vi "fit_fix height and width.vi"() -> ()   [LabVIEW 2016] (continued)
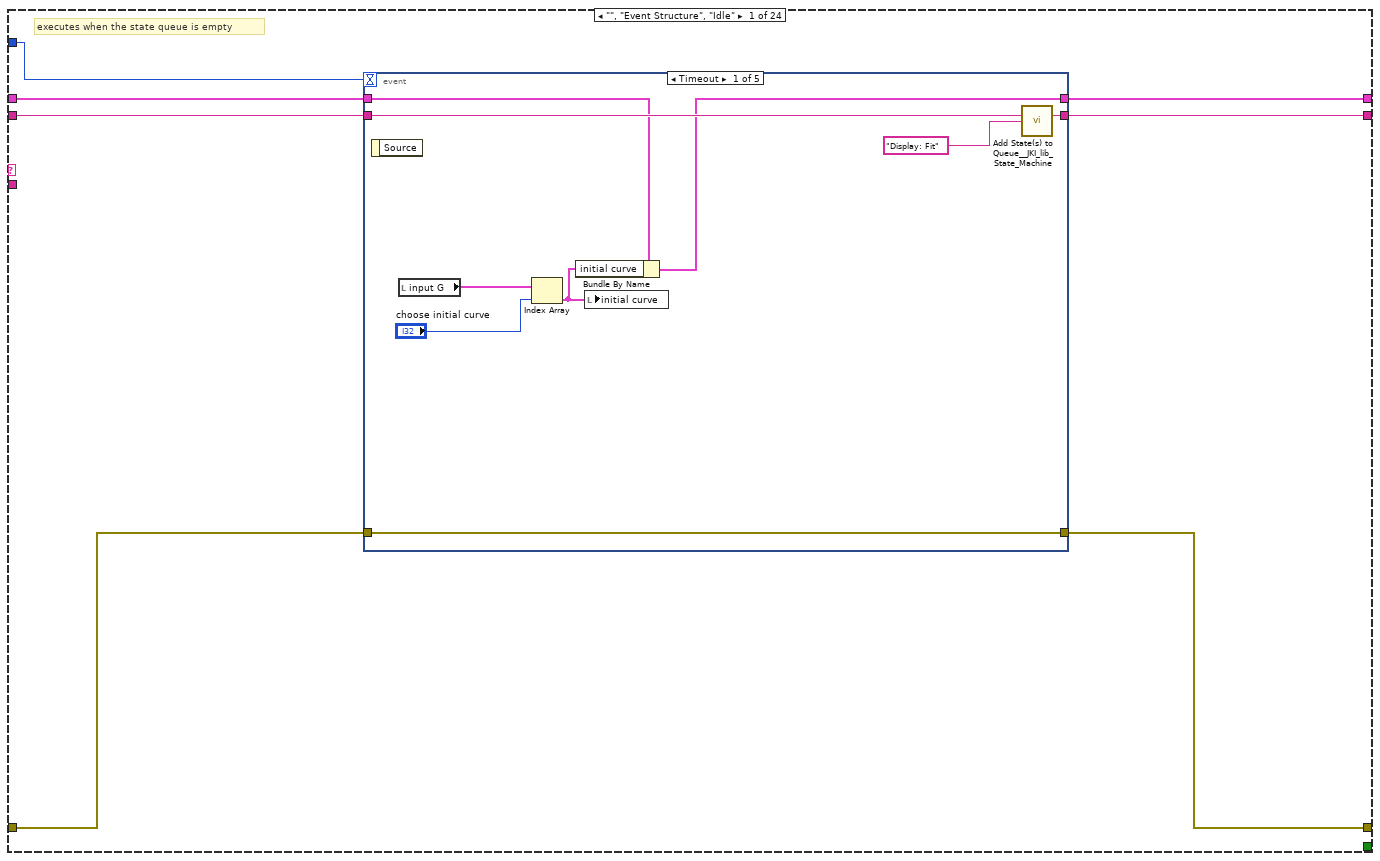
[diagram p3: hidden frame]
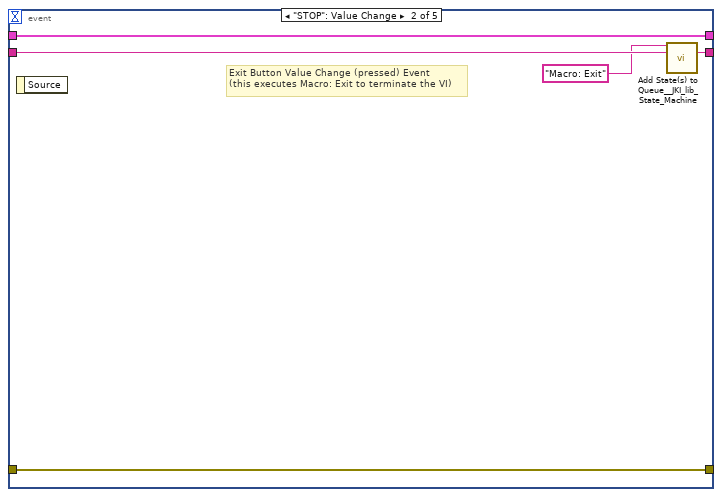
[diagram p4: hidden frame]
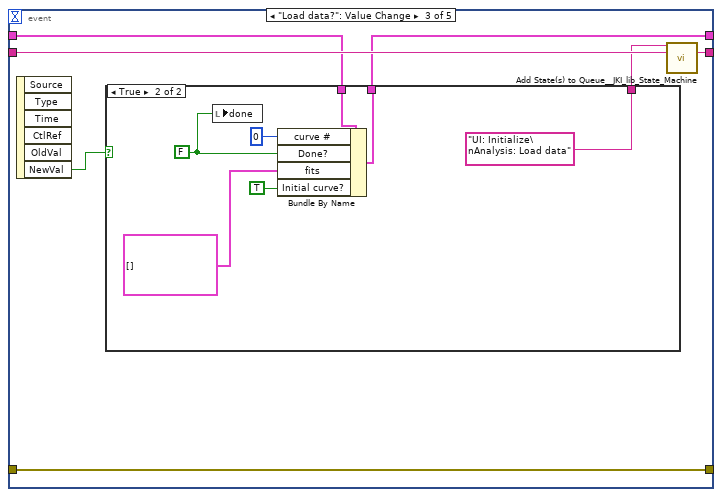
[diagram p5: hidden frame]
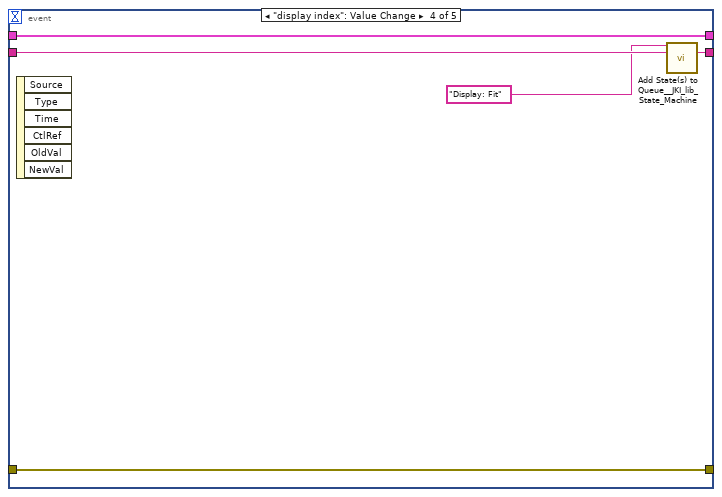
[diagram p7: hidden frame]
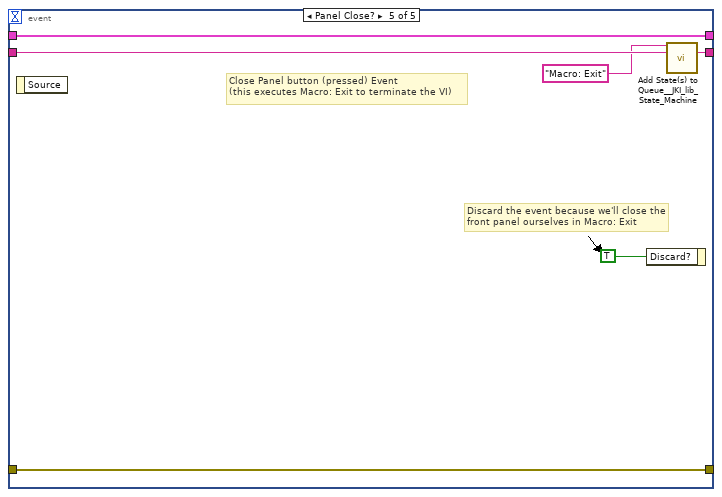
[diagram p8: hidden frame]
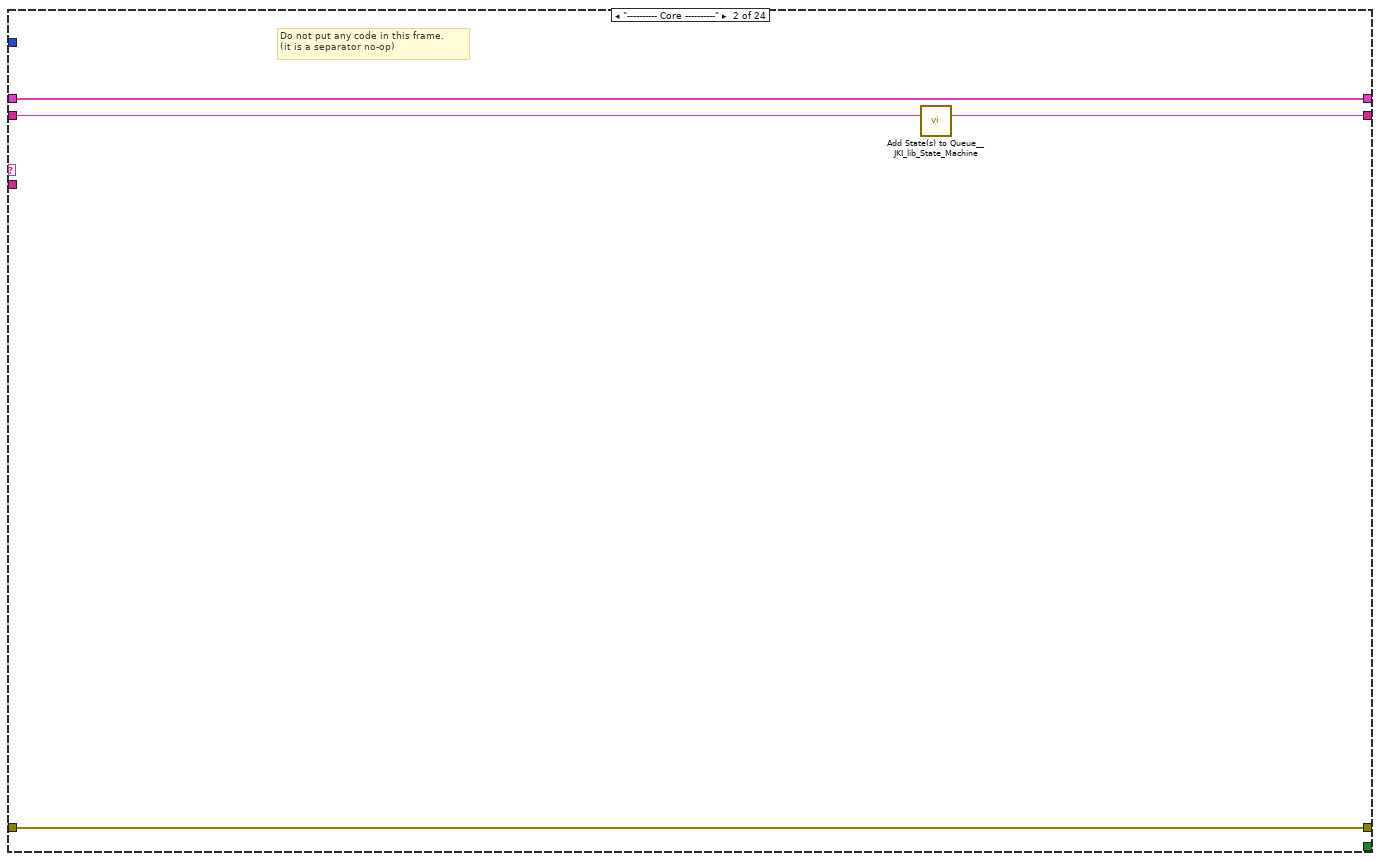
[diagram p9: hidden frame]
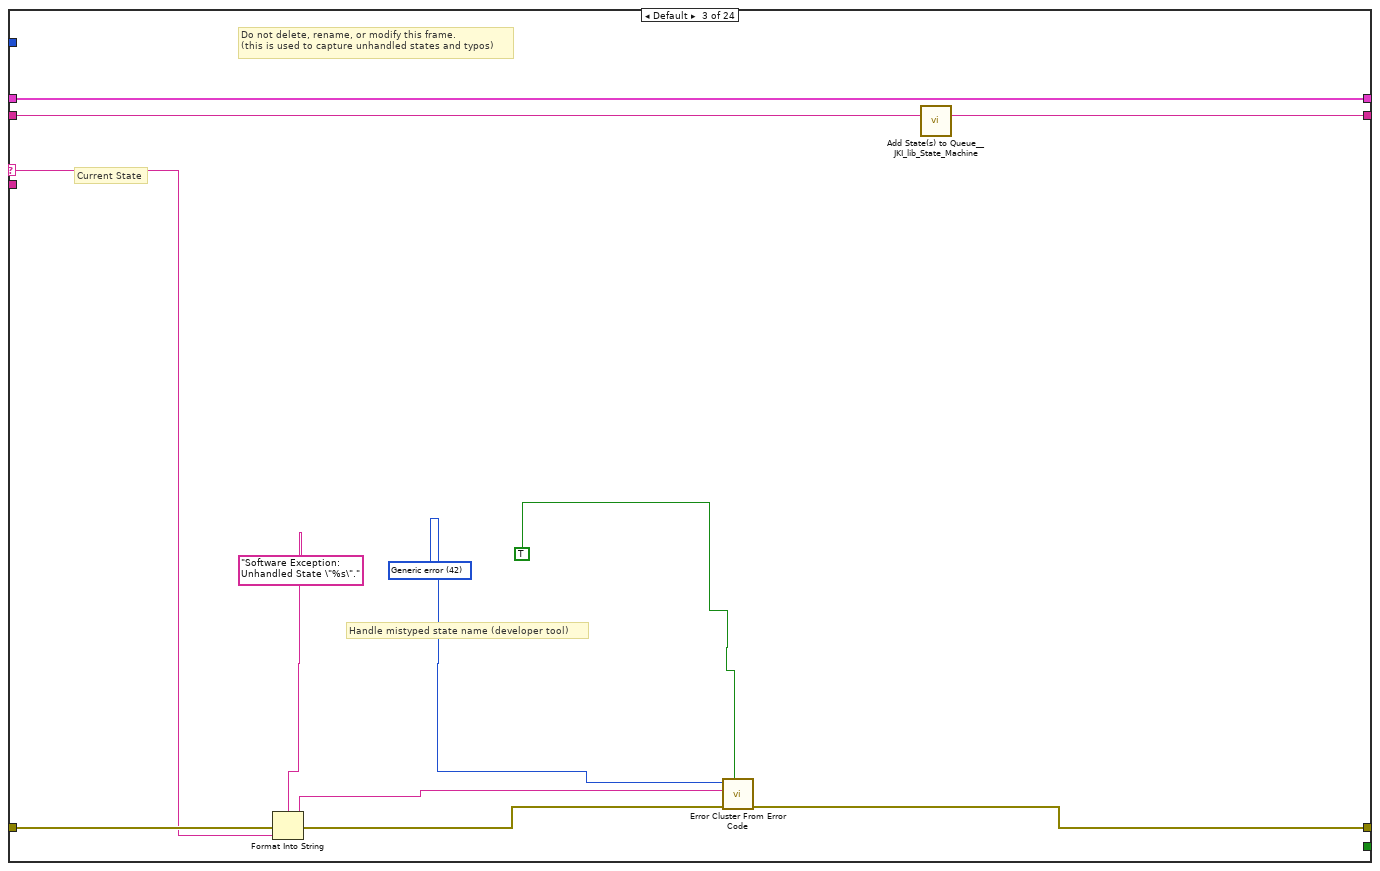
[diagram p10: hidden frame]
        n68 = call <vilib>:"Add State(s) to Queue__JKI_lib_State_Machine.vi"("State(s) in Front (\"\")"=w206, "State(s) in (\"\")"=w215) -> ("States Out"=w214:string)  [unwired: 13 in]
      }
      frame "---------- Analysis ----------" {
        # "Template Separator\n(You can make a copy of, or modify, this frame)"
        n69 = call <vilib>:"Add State(s) to Queue__JKI_lib_State_Machine.vi"("State(s) in (\"\")"=w219) -> ("States Out"=w218:string)  [unwired: 14 in]
      }
      frame "Analysis: Load data" {
        # "Load data and step through curves for fitting"
        n70 = local read "input G"() -> (w230:cluster{dbl[], dbl[]}[])
        n71 = Unbundle By Name(w243) -> ("curve #"=w229:i32, "fit iteration"=w225:i32, "Initial curve?"=w233:bool)
        "curve #" <- w229
        n72 = Array Size(array=w230) -> (size(s)=w228:i32)
        n73 = Decrement(x=w228) -> (x-1=w227:i32)
        n74 = case shown="True" "Restrict G?" {
          tunnel: w230 -> [w249 w251]
          tunnel: [w249 w250] -> w242
          frame False {
          }
          frame True {
            n75 = for {
              tunnel: w251 -> [w259] mode=indexing
              tunnel: [w252] -> w250 mode=indexing
              n76 = Unbundle(w259) -> (w257:dbl[], w256:dbl[])
              n77 = Threshold 1D Array(2:"Max G", 3:w256) -> (0:w255:dbl)  [unwired: 1 in]
              n78 = Array Subset(array=w256, length=w255) -> (w253:dbl[])  [unwired: 1 in]
              n79 = Array Subset(array=w257, length=w255) -> (w254:dbl[])  [unwired: 1 in]
              n80 = Bundle(w254, w253) -> (w252:cluster{dbl[], dbl[]})  [unwired: 1 in]
            }
          }
        }
        n81 = Equal?(x=w229, y=w227) -> (x = y?=w226:bool)
        n82 = Equal?(x=w225, y=0) -> (x = y?=w223:bool)
        n83 = And(x=w226, y=w223) -> (x .and. y?=w222:bool)
        n84 = local read "choose initial curve"() -> (w232:i32)
        n85 = case shown="True" w222 {
          frame False {
          }
          frame True {
            n86 = call <vilib>:"Beep.vi"() -> ()  [unwired: 12 in]
          }
        }
        n87 = Select(t=w232, s=w233, f=w229) -> (s? t:f=w231:i32)
        n88 = Index Array(array=w242, index=w231) -> (element=w234:cluster{dbl[], dbl[]})
        n89 = local write "Single G"(w234) -> ()
        n90 = local write "Restricted G"(w242) -> ()
        n91 = Unbundle(w234) -> (w240:dbl[])  [unwired: 1 out]
        n92 = Array Max & Min(array=w240) -> (max value=w241:dbl)  [unwired: 3 out]
        n93 = Round Toward -Infinity(1:w241) -> (0:w221:dbl)
        n94 = Add(x=w221, y=w225) -> (x+y=w239:dbl)
        n95 = Bundle By Name(cluster=w243, "All G"=w242, "Single G curve"=w234, "model step #"=w239) -> (w245:T5)
        n96 = Equal?(x=0, y=w225) -> (x = y?=w237:bool)
        n97 = Select(t="Analysis: find peaks" ("State(s) at Back (\"\")"), s=w237, f="Analysis: Initial Parameters" ("State(s) at Back (\"\")")) -> (s? t:f=w220:string)
        n98 = call <vilib>:"Add State(s) to Queue__JKI_lib_State_Machine.vi"("State(s) in Front (\"\")"=w220, "State(s) in (\"\")"=w248) -> ("States Out"=w247:string)  [unwired: 13 in]
      }
      frame "Analysis: find peaks" {
        # "Fid peak locations to help constrain step position inital parameters"
        n99 = Unbundle By Name(w271) -> ("Single G curve"=w272:cluster{"Single G curve":dbl[], dbl[]})
        n100 = call <userlib>:"differential.vi"("Numeric"="derivative \nfor peak initial conditions", "dy/dx vs x"=TRUE, "A vs B 2"=w272) -> ("A vs B 3"=w267:T8)  [unwired: 1 in]
        n101 = Unbundle(w267) -> ("Decimated Array"=w263:dbl[], "Decimated Array"=w266:dbl[])
        n102 = call <vilib>:"Peak Detector.vi"("width"="derivative peak width", "threshold"="derivative peak threshold", "X"=w266) -> ("Locations"=w262:dbl[])  [unwired: 4 in, 4 out]
        "Locations index" <- w262
        n103 = for {
          N -> [w276]
          tunnel: w263 -> [w279]
          tunnel: w262 -> [w278] mode=indexing
          tunnel: [w277] -> w261 mode=indexing
          tunnel: [w276] -> _ mode=indexing
          n104 = Interpolate 1D Array(1:w278, 2:w279) -> (0:w277:dbl)
        }
        "Locations" <- w261
        n105 = call <vilib>:"Add State(s) to Queue__JKI_lib_State_Machine.vi"("State(s) in Front (\"\")"="Analysis: Initial Parameters" ("State(s) at Back (\"\")"), "State(s) in (\"\")"=w275) -> ("States Out"=w274:string)  [unwired: 13 in]
        n106 = Bundle By Name(cluster=w271, "Locations index"=w262, "Locations"=w261) -> (w270:T5)
      }
      frame "Analysis: Initial Parameters" {
        # "Create initial parameter and parameter bound arrays"
        n107 = Unbundle By Name(w306) -> ("Initial Best Fit"=w297:dbl[], "Initial curve?"=w288:bool, "model step #"=w301:i32, "Single G curve"=w309:cluster{"Single G curve":dbl[], dbl[]}, "Locations index"=w308:dbl[], "Locations"=w307:dbl[], "Best Fit Parameters"=w292:dbl[][], "residues"=w291:dbl[], "curve #"=w281:i32)
        n108 = case shown="True" "fix step width?" {
          tunnel: [w315 w316] -> w296
          tunnel: [w314 w316] -> w295
          tunnel: ["step width?" w316] -> w284
          tunnel: w281 -> [_ w324]
          frame False {
            n109 = local read "step width max"() -> (w315:dbl)
            n110 = local read "step width min"() -> (w314:dbl)
          }
          frame True {
            n111 = local read "B multiplier"() -> (w323:dbl)
            n112 = local read "B offset"() -> (w321:dbl)
            n113 = Multiply(x=w324, y=w323) -> (x*y=w322:dbl)
            n114 = Add(x=w322, y=w321) -> (x+y=w319:dbl)
            n115 = Multiply(x=w319, y="fix width slope") -> (x*y=w317:dbl)
            n116 = Add(x=w317, y="fix width intercept") -> (x+y=w316:dbl)
          }
        }
        n117 = Array Size(array=w291) -> (size(s)=w290:i32)
        n118 = Unbundle(w309) -> ("Single G curve"=w302:dbl[], w303:dbl[])
        n119 = Select(t=w288, s="fit inital parameters?", f=TRUE) -> (s? t:f=w287:bool)
        n120 = Decrement(x=w290) -> (x-1=w289:i32)
        n121 = case shown="True" w287 {
          tunnel: w308 -> [w339 w400]
          tunnel: w307 -> [w338 w399]
          tunnel: [w347 w398] -> w305
          tunnel: w303 -> [w341 w397]
          tunnel: w302 -> [w344 w396]
          tunnel: w301 -> [w351 w395]
          tunnel: [w337 w394] -> w300
          tunnel: [w345 w393] -> w299
          tunnel: w297 -> [w348 _]
          tunnel: w296 -> [w336 w392]
          tunnel: w295 -> [w335 w391]
          tunnel: "step height max" -> [w334 w390]
          tunnel: "step height min" -> [w333 w389]
          tunnel: w292 -> [w332 _]
          tunnel: w289 -> [w331 _]
          tunnel: "one width?" -> [_ w388]
          tunnel: w284 -> [_ w387]
          frame False {
            w346 = dbl[] []
            n122 = Index Array(array=w332, index (row)=w331) -> (element=w330:dbl[])  [unwired: 1 in]
            n123 = Array Max & Min(array=w344) -> (max value=w343:dbl, min value=w342:dbl)  [unwired: 2 out]
            n124 = call-poly <userlib>:"Filter 1D Array__ogtk.vi"("items to filter"=0.0, "array"=w348) -> ("filtered array"=w352:dbl[])  [unwired: 4 in, 1 out]
            n125 = Decimate 1D Array(w330) -> (w328:dbl[])  [unwired: 2 out]
            n126 = Multiply(x=w328, y="Max position %") -> (x*y=w326:dbl[])
            n127 = Multiply(x=w328, y="Min position %") -> (x*y=w325:dbl[])
            n128 = Decimate 1D Array(w352) -> (w350:dbl[], w349:dbl[])  [unwired: 1 out]
            n129 = for {
              N: w351 -> [_]
              tunnel: w350 -> [w386]
              tunnel: w349 -> [w385]
              shift-right: [w383] -> w347
              shift-left: dbl[] [] -> [w384]
              shift-right: [w381] -> w345
              shift-left: w346 -> [w382]
              shift-right: [w379] -> w337
              shift-left: w346 -> [w380]
              tunnel: w343 -> [w371]
              tunnel: w342 -> [w368]
              tunnel: w341 -> [w378]
              tunnel: w339 -> [w377]
              tunnel: w338 -> [w375]
              tunnel: w336 -> [w360]
              tunnel: w335 -> [w359]
              tunnel: w334 -> [w362]
              tunnel: w333 -> [w361]
              tunnel: w326 -> [w367]
              tunnel: w325 -> [w365]
              i -> [w364]
              n130 = Index Array(array=w367, index=w364) -> (element=w366:dbl)
              n131 = Index Array(array=w365, index=w364) -> (element=w363:dbl)
              n132 = Index Array(array=w386, index=w364) -> (element=w356:dbl)
              n133 = Index Array(array=w385, index=w364) -> (element=w372:dbl)
              n134 = Threshold 1D Array(2:w364, 3:w378) -> (0:w376:dbl)  [unwired: 1 in]
              n135 = call "compare if zero.vi"("if zero out"=w368, "Numeric"=w363) -> ("out"=w369:dbl)  [unwired: 5 in]
              n136 = call "compare if zero.vi"("if zero out"=w362, "Numeric"=w356) -> ("out"=w358:dbl)  [unwired: 5 in]
              n137 = call "compare if zero.vi"("if zero out"=w371, "Numeric"=w366) -> ("out"=w370:dbl)  [unwired: 5 in]
              n138 = call "Search 1D Array for Nearest LV2012 NIVerified.vi"("desired element"=w376, "1D Array"=w377) -> ("closest index"=w374:i32)  [unwired: 8 in, 1 out]
              n139 = call "compare if zero.vi"("if zero out"=w360, "Numeric"=w372) -> ("out"=w355:dbl)  [unwired: 5 in]
              n140 = call "compare if zero.vi"("if zero out"=w361, "Numeric"=w356) -> ("out"=w357:dbl)  [unwired: 5 in]
              n141 = call "compare if zero.vi"("if zero out"=w359, "Numeric"=w372) -> ("out"=w354:dbl)  [unwired: 5 in]
              n142 = Index Array(array=w375, index=w374) -> (element=w373:dbl)
              n143 = Build Array (concatenate)(w382, w358, w370, w355) -> (w381:dbl[])
              n144 = Build Array (concatenate)(w380, w357, w369, w354) -> (w379:dbl[])
              n145 = Build Array (concatenate)(w384, w356, w373, w372) -> (w383:dbl[])
            }
          }
          frame True {
            n146 = case shown="True" w388 {
              tunnel: w400 -> [w418 w453]
              tunnel: w399 -> [w417 w452]
              tunnel: [w416 w451] -> w398
              tunnel: w397 -> [w415 w450]
              tunnel: w396 -> [w414 w448]
              tunnel: w395 -> [w411 w445]
              tunnel: [w410 w444] -> w394
              tunnel: [w409 w443] -> w393
              tunnel: w392 -> [w404 w441]
              tunnel: w391 -> [w402 w440]
              tunnel: w390 -> [w408 w439]
              tunnel: w389 -> [w407 w438]
              tunnel: w387 -> [w406 w437]
              frame True {
                n147 = Array Max & Min(array=w414) -> (max value=w413:dbl, min value=w412:dbl)  [unwired: 2 out]
                n148 = Build Array(w406) -> (w405:dbl[])
                n149 = Build Array(w404) -> (w403:dbl[])
                n150 = Build Array(w402) -> (w401:dbl[])
                n151 = for {
                  N: w411 -> [_]
                  tunnel: w415 -> [w436]
                  shift-right: [w428] -> w416
                  shift-left: w405 -> [w429]
                  tunnel: w418 -> [w434]
                  tunnel: w417 -> [w432]
                  shift-right: [w426] -> w409
                  shift-left: w403 -> [w427]
                  shift-right: [w425] -> w410
                  shift-left: w401 -> [w424]
                  tunnel: w413 -> [w423]
                  tunnel: w412 -> [w421]
                  tunnel: w404 -> [_]
                  tunnel: w402 -> [_]
                  tunnel: w408 -> [w420]
                  tunnel: w407 -> [w419]
                  i -> [w435]
                  n152 = Threshold 1D Array(2:w435, 3:w436) -> (0:w433:dbl)  [unwired: 1 in]
                  n153 = call "Search 1D Array for Nearest LV2012 NIVerified.vi"("desired element"=w433, "1D Array"=w434) -> ("closest index"=w422:i32)  [unwired: 8 in, 1 out]
                  n154 = Index Array(array=w432, index=w422) -> (element=w430:dbl)
                  n155 = Build Array (concatenate)(w429, 1.0 ("element"), w430) -> (w428:dbl[])
                  n156 = Build Array (concatenate)(w427, w420, w423) -> (w426:dbl[])
                  n157 = Build Array (concatenate)(w424, w419, w421) -> (w425:dbl[])
                }
              }
              frame False {
                w442 = dbl[] []
                n158 = Array Max & Min(array=w448) -> (max value=w447:dbl, min value=w446:dbl)  [unwired: 2 out]
                n159 = for {
                  N: w445 -> [_]
                  tunnel: w450 -> [w474]
                  shift-right: [w466] -> w451
                  shift-left: dbl[] [] -> [w467]
                  tunnel: w453 -> [w472]
                  tunnel: w452 -> [w470]
                  shift-right: [w464] -> w443
                  shift-left: w442 -> [w465]
                  shift-right: [w463] -> w444
                  shift-left: w442 -> [w462]
                  tunnel: w447 -> [w461]
                  tunnel: w446 -> [w459]
                  tunnel: w441 -> [w458]
                  tunnel: w440 -> [w457]
                  tunnel: w439 -> [w456]
                  tunnel: w438 -> [w455]
                  tunnel: w437 -> [w454]
                  i -> [w473]
                  n160 = Threshold 1D Array(2:w473, 3:w474) -> (0:w471:dbl)  [unwired: 1 in]
                  n161 = call "Search 1D Array for Nearest LV2012 NIVerified.vi"("desired element"=w471, "1D Array"=w472) -> ("closest index"=w460:i32)  [unwired: 8 in, 1 out]
                  n162 = Index Array(array=w470, index=w460) -> (element=w468:dbl)
                  n163 = Build Array (concatenate)(w467, 1.0 ("element"), w468, w454) -> (w466:dbl[])
                  n164 = Build Array (concatenate)(w465, w456, w461, w458) -> (w464:dbl[])
                  n165 = Build Array (concatenate)(w462, w455, w459, w457) -> (w463:dbl[])
                }
              }
            }
          }
        }
        "Initial Parameters" <- w305
        n166 = Bundle(w300, w299) -> (w298:cluster{dbl[], dbl[]})  [unwired: 1 in]
        n167 = call <vilib>:"Add State(s) to Queue__JKI_lib_State_Machine.vi"("State(s) in Front (\"\")"="Analysis: Fit" ("State(s) at Back (\"\")"), "State(s) in (\"\")"=w312) -> ("States Out"=w311:string)  [unwired: 13 in]
        n168 = Bundle By Name(cluster=w306, "Initial Parameters"=w305, "parameter bounds"=w298, "one width?"="one width?") -> (w304:T5)
      }
      frame "Analysis: Fit" {
        (unwired) errorcluster {"status"=FALSE, "code"=0, "source"=""} ("error out")
        # "increase termination conditions \nif there is a max iteration error"
        # "Fit data"
        n169 = Unbundle By Name(w511) -> ("termination"=w498:cluster{"max iteration":i32, "tolerance":dbl}, "intermediate fits"=w501:cluster{dbl[], dbl[]}[], "Single G curve"=w508:cluster{"Single G curve":dbl[], dbl[]}, "Initial Parameters"=w515:dbl[], "Intermediate Best Fit"=w509:dbl[][], "intermediate residues"=w504:dbl[], "termination"=w506:cluster{"max iteration":i32, "tolerance":dbl}, "parameter bounds"=w507:T6, "Intermediate delta"=w484:dbl[][])
        "termination" <- w506
        n170 = case shown="\"normal tanh\", Default" "fit vi path" {
          tunnel: [path "C:/user/megan/hg/levylab_user_megan/data analysis/pascal fitting/subVI/LM model function and gradient_step.vi" ("vi path") path "C:/user/megan/hg/levylab_user_megan/data analysis/pascal fitting/subVI/LM model function_1 width.vi" ("vi path")] -> w485
          frame "normal tanh", Default {
          }
          frame "tanh w/ 1 width" {
          }
        }
        n171 = Unbundle(w508) -> ("Single G curve"=w481:dbl[], w482:dbl[])
        n172 = Open VI Reference(type specifier VI Refnum (for type only)=refnum<vi> refnum, vi path=w485) -> (vi reference=w512:refnum<vi>)  [unwired: 4 in, 1 out]
        n173 = call-by-ref "?"(reference=w512, "X"=w481, "a"=w515) -> (reference out=w479:refnum<vi>)  [unwired: 3 in, 4 out]
        n174 = Unbundle(w498) -> ("max iteration"=w497:i32, "tolerance"=w496:dbl)
        n175 = call-poly <vilib>:"Constrained Nonlinear Curve Fit.vi"("Y"=w482, "f(x,a)"=w479, "X"=w481, "initial parameters"=w515, "error in (no error)"=w510, "termination"=w506, "parameter bounds"=w507, "method"="method") -> ("best nonlinear fit"=w491:dbl[], "best fit parameters"=w480:dbl[], "residue"=w487:dbl, "error out"=w477:errorcluster)  [unwired: 2 in, 2 out]
        n176 = call <vilib>:"Goodness of Fit.vi"("Best Fit"=w491, "Y"=w482) -> ("RMSE"=→"RMSE":dbl, "R-square"=→"R-square":dbl, "SSE"=→"SSE":dbl)  [unwired: 6 in, 1 out]
        n177 = disable-structure shown="Disabled" {
          disable-tunnel: w482 -> [w523 _]
          disable-tunnel: w481 -> [w522 _]
          disable-tunnel: w480 -> [w521 _]
          disable-tunnel: w479 -> [w520 _]
          disable-tunnel: [w519 _] -> w478
          disable-tunnel: w477 -> [w518 _]
          frame Disabled {
            n178 = call <vilib>:"Nonlinear Curve Fit Intervals.vi"("Y"=w523, "f(x,a)"=w520, "X"=w522, "best fit parameters"=w521, "error in (no error)"=w518) -> ("delta best fit parameters"=w519:dbl[])  [unwired: 7 in, 3 out]
          }
          frame Enabled {
          }
        }
        n179 = Bundle("Single G curve"=w481, "best nonlinear fit"=w491) -> (w502:T9)  [unwired: 1 in]
        n180 = Equal?(x=errorcluster {"status"=TRUE, "code"=-23026, "source"="maximum iterations exceeded"} ("error out"), y=w477) -> (x = y?=w499:bool)
        n181 = case shown="True" w499 {
          tunnel: w509 -> [w541 w553]
          tunnel: w480 -> [w540 _]
          tunnel: [w539 w553] -> w505
          tunnel: w504 -> [w538 w552]
          tunnel: w487 -> [w537 _]
          tunnel: [w536 w552] -> w503
          tunnel: w502 -> [w535 _]
          tunnel: [w534 w551] -> w500
          tunnel: w501 -> [w533 w551]
          tunnel: w497 -> [w532 w547]
          tunnel: w496 -> [w531 w548]
          tunnel: [w531 w546] -> w494
          tunnel: [w532 w545] -> w495
          tunnel: ["Analysis: Iterate" "Analysis: Fit"] -> w475
          tunnel: w477 -> [w527 _]
          tunnel: [w527 errorcluster {"status"=FALSE, "code"=0, "source"=""} ("error out")] -> w493
          tunnel: w484 -> [w529 w542]
          tunnel: [w528 w542] -> w483
          tunnel: w480 -> [_ _]
          tunnel: w481 -> [_ _]
          tunnel: w482 -> [_ _]
          tunnel: w479 -> [_ _]
          tunnel: w478 -> [w526 _]
          frame False {
            n182 = Build Array (concatenate)(w541, w540) -> (w539:dbl[][])
            n183 = Build Array (concatenate)(w538, w537) -> (w536:dbl[])
            n184 = Build Array (concatenate)(w529, w526) -> (w528:dbl[][])
            n185 = Insert Into Array(array=w533, new element=w535) -> (w534:cluster{dbl[], dbl[]}[])  [unwired: 1 in]
          }
          frame True {
            n186 = Multiply(x=w548, y=2.0) -> (x*y=w546:dbl)
            n187 = Add(x=w547, y=200) -> (x+y=w545:i32)
          }
        }
        "intermediate residues" <- w503
        "Intermediate Best Fit" <- w505
        n188 = Bundle By Name(cluster=w511, "termination.max iteration"=w495, "termination.tolerance"=w494, "intermediate fits"=w500, "Intermediate Best Fit"=w505, "intermediate residues"=w503, "Intermediate delta"=w483) -> (w514:T5)
        n189 = call <vilib>:"Add State(s) to Queue__JKI_lib_State_Machine.vi"("State(s) in Front (\"\")"=w475, "State(s) in (\"\")"=w517) -> ("States Out"=w516:string)  [unwired: 13 in]
      }
      frame "Analysis: Iterate" {
        # "Iterate curve # and fit iteration #\nincrement fit iteration\nif fit iteration = 3, set to 0 and increment curve #\nif curve # is greater than the total # of curves end fitting"
        n190 = Unbundle By Name(w590) -> ("curve #"=w585:i32, "All G"=w584:cluster{dbl[], dbl[]}[], "fit iteration"=w588:i32, "Best Fit Parameters"=w579:dbl[][], "Intermediate Best Fit"=w581:dbl[][], "intermediate residues"=w580:dbl[], "residues"=w573:dbl[], "Intermediate delta"=w559:dbl[][], "delta best fit"=w556:dbl[][], "fits"=w560:cluster{dbl[], dbl[]}[], "intermediate fits"=w575:cluster{dbl[], dbl[]}[], "Initial curve?"=w571:bool, "Initial Best Fit"=w569:dbl[], "All locations"=w567:dbl[][], "Locations"=w568:dbl[], "Fit steps"=w564:i32[], "model step #"=w563:i32)
        n191 = Increment(x=w588) -> (x+1=w587:i32)
        n192 = case shown="4" w587 {
          selector: w587 -> [w608 _]
          tunnel: [w608 0] -> w586
          tunnel: w585 -> [w607 w624]
          tunnel: w584 -> [_ w651]
          tunnel: [w607 w647] -> w583
          tunnel: ["Analysis: Load data" w646] -> w554
          tunnel: w581 -> [w603 w622]
          tunnel: w580 -> [w605 w645]
          tunnel: w579 -> [w604 w644]
          tunnel: [w604 w643] -> w576
          tunnel: [w603 w612] -> w578
          tunnel: [w605 dbl[] [] ("residues")] -> w577
          tunnel: w560 -> [w602 w640]
          tunnel: w575 -> [w601 w641]
          tunnel: [w602 w638] -> w574
          tunnel: [w601 cluster{dbl[], dbl[]}[] [] ("intermediate fits")] -> w558
          tunnel: w573 -> [w600 w636]
          tunnel: [w600 w634] -> w572
          tunnel: w571 -> [w599 w632]
          tunnel: [w599 FALSE] -> w570
          tunnel: [w598 w631] -> w562
          tunnel: w569 -> [w598 w630]
          tunnel: w568 -> [_ w627]
          tunnel: w567 -> [w597 w628]
          tunnel: [w597 w626] -> w566
          tunnel: w564 -> [w596 w625]
          tunnel: [w596 w623] -> w565
          tunnel: w563 -> [_ _]
          tunnel: w559 -> [w595 w615]
          tunnel: [w595 w612] -> w557
          tunnel: w556 -> [w594 w613]
          tunnel: [w594 w611] -> w555
          frame 0, Default {
          }
          frame 4 {
            w612 = dbl[][] [] ("Intermediate Best Fit")
            n193 = Increment(x=w624) -> (x+1=w648:i32)
            n194 = Array Size(array=w651) -> (size(s)=w649:i32)
            n195 = Array Max & Min(array=w645) -> (min value=w635:dbl, min index (indices)=w614:i32)  [unwired: 2 out]
            n196 = Less?(x=w648, y=w649) -> (x < y?=w650:bool)
            n197 = Index Array(array=w641, index=w614) -> (element=w639:cluster{dbl[], dbl[]})
            n198 = Index Array(array=w622, index (row)=w614) -> (element=w618:dbl[])  [unwired: 1 in]
            n199 = Index Array(array=w615, index (row)=w614) -> (element=w610:dbl[])  [unwired: 1 in]
            n200 = case shown="True" w632 {
              tunnel: w618 -> [w654 w657]
              tunnel: [w655 w657] -> w631
              tunnel: w630 -> [w655 _]
              tunnel: [w654 w656] -> w629
              tunnel: w610 -> [w653 _]
              tunnel: [w653 w656] -> w609
              frame False {
              }
              frame True {
                w656 = dbl[] [] ("residues")
              }
            }
            n201 = case shown="True" w650 {
              tunnel: w648 -> [_ w660]
              tunnel: [0 w660] -> w647
              tunnel: ["Display: Fit" "Analysis: Load data"] -> w646
              frame False {
              }
              frame True {
              }
            }
            n202 = call-poly <userlib>:"Filter 1D Array__ogtk.vi"("items to filter"=0, "array"=w618) -> ("filtered array"=w617:dbl[])  [unwired: 4 in, 1 out]
            n203 = Build Array (concatenate)(w628, w627) -> (w626:dbl[][])
            n204 = Build Array (concatenate)(w636, w635) -> (w634:dbl[])
            n205 = Array Size(array=w617) -> (size(s)=w621:i32)
            n206 = Build Array (concatenate)(w640, w639) -> (w638:cluster{dbl[], dbl[]}[])
            n207 = Build Array (concatenate)(w613, w609) -> (w611:dbl[][])
            n208 = Divide(x=w621, y=3) -> (x/y=w619:dbl)
            n209 = Build Array (concatenate)(w644, w629) -> (w643:dbl[][])
            n210 = Build Array (concatenate)(w625, w619) -> (w623:dbl[])
          }
        }
        "Best Fit Parameters" <- w576
        "residues" <- w572
        "Initial Best Fit" <- w562
        "Fit steps" <- w565
        "delta best fit" <- w555
        n211 = call <vilib>:"Add State(s) to Queue__JKI_lib_State_Machine.vi"("State(s) in Front (\"\")"=w554, "State(s) in (\"\")"=w593) -> ("States Out"=w592:string)  [unwired: 13 in]
        n212 = local write "fits"(w574) -> ()
        n213 = call "parse best fit into string array.vi"("Initial Best Fit"=w562) -> ("concatenated string"=→"initial best fit":string)  [unwired: 10 in]
        n214 = Bundle By Name(cluster=w590, "curve #"=w583, "fit iteration"=w586, "termination"=cluster{"max iteration":i32, "tolerance":dbl} {"max iteration"=200, "tolerance"=1e-08}, "Best Fit Parameters"=w576, "Intermediate Best Fit"=w578, "intermediate residues"=w577, "residues"=w572, "Intermediate delta"=w557, "delta best fit"=w555, "intermediate fits"=w558, "fits"=w574, "Initial curve?"=w570, "Initial Best Fit"=w562, "All locations"=w566, "Fit steps"=w565) -> (w591:T5)
      }
      frame "----------Display-------------" {
        # "Your code here.\n(You can make a copy of, or modify, this frame)"
        n215 = call <vilib>:"Add State(s) to Queue__JKI_lib_State_Machine.vi"("State(s) in (\"\")"=w665) -> ("States Out"=w664:string)  [unwired: 14 in]
      }
      frame "Display: Fit" {
        # "place holder for B field values"
        # "extract and sort Vsg peak values"
        n216 = Unbundle By Name(w723) -> ("All G"=w721:cluster{dbl[], dbl[]}[], "fits"=w716:cluster{dbl[], dbl[]}[], "Best Fit Parameters"=w714:dbl[][], "residues"=w713:dbl[], "one width?"=w670:bool, "delta best fit"=w669:dbl[][])  [unwired: 1 out]
        n217 = Index Array(array=w713, index="display index") -> (element=→"Display residue":dbl)
        n218 = Array Size(array=w713) -> (size(s)=w712:i32)
        n219 = for {
          N: w712 -> [_]
          tunnel: [w804] -> w667 mode=indexing
          i -> [w806]
          n220 = local read "B multiplier"() -> (w802:dbl)
          n221 = local read "B offset"() -> (w803:dbl)
          n222 = Multiply(x=w802, y=w806) -> (x*y=w805:dbl)
          n223 = Add(x=w803, y=w805) -> (x+y=w804:dbl)
        }
        n224 = case shown="False" w670 {
          tunnel: [w733 w765] -> w715
          tunnel: w714 -> [w732 w764]
          tunnel: w712 -> [w731 w763]
          tunnel: [w730 w762] -> w681
          tunnel: [w729 w761] -> w679
          tunnel: w669 -> [w728 w760]
          tunnel: [w727 w759] -> w668
          frame False {
            n225 = for {
              N: w731 -> [_]
              tunnel: w732 -> [w758]
              tunnel: [w751] -> w733 mode=indexing
              tunnel: [w748] -> w730 mode=indexing
              tunnel: [w746] -> w729 mode=indexing
              tunnel: w728 -> [w745]
              tunnel: [w734] -> w727 mode=indexing
              i -> [w744]
              w742 = 0.0
              w753 = 0.0
              n226 = Index Array(array=w758, index (row)=w744) -> (element=w757:dbl[])  [unwired: 1 in]
              n227 = Index Array(array=w745, index (row)=w744) -> (element=w743:dbl[])  [unwired: 1 in]
              n228 = Decimate 1D Array(w757) -> (w755:dbl[], w756:dbl[], w754:dbl[])
              n229 = Decimate 1D Array(w743) -> (w741:dbl[], w740:dbl[], w739:dbl[])
              n230 = call-poly <userlib>:"Filter 1D Array__ogtk.vi"("items to filter"=w742, "array"=w739) -> ("filtered array"=w737:dbl[])  [unwired: 4 in, 1 out]
              n231 = call-poly <userlib>:"Filter 1D Array__ogtk.vi"("items to filter"=w753, "array"=w754) -> ("filtered array"=w747:dbl[])  [unwired: 4 in, 1 out]
              n232 = call-poly <userlib>:"Filter 1D Array__ogtk.vi"("items to filter"=w742, "array"=w741) -> ("filtered array"=w735:dbl[])  [unwired: 4 in, 1 out]
              n233 = call-poly <userlib>:"Filter 1D Array__ogtk.vi"("items to filter"=w742, "array"=w740) -> ("filtered array"=w736:dbl[])  [unwired: 4 in, 1 out]
              n234 = call-poly <userlib>:"Filter 1D Array__ogtk.vi"("items to filter"=w753, "array"=w756) -> ("filtered array"=w752:dbl[])  [unwired: 4 in, 1 out]
              n235 = call-poly <userlib>:"Filter 1D Array__ogtk.vi"("items to filter"=w753, "array"=w755) -> ("filtered array"=w749:dbl[])  [unwired: 4 in, 1 out]
              n236 = call-poly <userlib>:"Sort Array__ogtk.vi"("Order"=enum16{"ascending", "descending"}."ascending", "Array in"=w752) -> ("Sorted Pointers"=w738:i32[], "Sorted Array out"=w751:dbl[])  [unwired: 8 in]
              n237 = call-poly <userlib>:"Reorder Array2__ogtk.vi"("indices"=w738, "array"=w735) -> ()  [unwired: 9 in, 1 out]
              n238 = call-poly <userlib>:"Reorder Array2__ogtk.vi"("indices"=w738, "array"=w736) -> ("reordered array"=w734:dbl[])  [unwired: 9 in]
              n239 = call-poly <userlib>:"Reorder Array2__ogtk.vi"("indices"=w738, "array"=w737) -> ()  [unwired: 9 in, 1 out]
              n240 = call-poly <userlib>:"Reorder Array2__ogtk.vi"("indices"=w738, "array"=w747) -> ("reordered array"=w746:dbl[])  [unwired: 9 in]
              n241 = call-poly <userlib>:"Reorder Array2__ogtk.vi"("indices"=w738, "array"=w749) -> ("reordered array"=w748:dbl[])  [unwired: 9 in]
            }
          }
          frame True {
            n242 = for {
              N: w763 -> [_]
              tunnel: w764 -> [w792]
              tunnel: [w775] -> w765 mode=indexing
              tunnel: [w774] -> w762 mode=indexing
              tunnel: [w784] -> w761 mode=indexing
              tunnel: w760 -> [w783]
              tunnel: [w766] -> w759 mode=indexing
              i -> [w782]
              w770 = 0.0
              w789 = 0.0
              n243 = Index Array(array=w783, index (row)=w782) -> (element=w781:dbl[])  [unwired: 1 in]
              n244 = Index Array(array=w792, index (row)=w782) -> (element=w788:dbl[])  [unwired: 1 in]
              n245 = Delete From Array(array=w788, length=1, index=0) -> (deleted portion=w784:dbl[], array with subset deleted=w785:dbl[])
              n246 = Delete From Array(array=w781, length=1, index=0) -> (array with subset deleted=w778:dbl[])  [unwired: 1 out]
              n247 = Decimate 1D Array(w785) -> (w790:dbl[], w791:dbl[])
              n248 = Decimate 1D Array(w778) -> (w772:dbl[], w771:dbl[])
              n249 = call-poly <userlib>:"Filter 1D Array__ogtk.vi"("items to filter"=w789, "array"=w791) -> ("filtered array"=w777:dbl[])  [unwired: 4 in, 1 out]
              n250 = call-poly <userlib>:"Filter 1D Array__ogtk.vi"("items to filter"=w789, "array"=w790) -> ("filtered array"=w776:dbl[])  [unwired: 4 in, 1 out]
              n251 = call-poly <userlib>:"Filter 1D Array__ogtk.vi"("items to filter"=w770, "array"=w772) -> ("filtered array"=w769:dbl[])  [unwired: 4 in, 1 out]
              n252 = call-poly <userlib>:"Filter 1D Array__ogtk.vi"("items to filter"=w770, "array"=w771) -> ("filtered array"=w768:dbl[])  [unwired: 4 in, 1 out]
              n253 = call-poly <userlib>:"Sort Array__ogtk.vi"("Order"=enum16{"ascending", "descending"}."ascending", "Array in"=w777) -> ("Sorted Pointers"=w767:i32[], "Sorted Array out"=w775:dbl[])  [unwired: 8 in]
              n254 = call-poly <userlib>:"Reorder Array2__ogtk.vi"("indices"=w767, "array"=w776) -> ("reordered array"=w774:dbl[])  [unwired: 9 in]
              n255 = call-poly <userlib>:"Reorder Array2__ogtk.vi"("indices"=w767, "array"=w769) -> ()  [unwired: 9 in, 1 out]
              n256 = call-poly <userlib>:"Reorder Array2__ogtk.vi"("indices"=w767, "array"=w768) -> ("reordered array"=w766:dbl[])  [unwired: 9 in]
            }
          }
        }
        n257 = Index Array(array=w714, index (row)="display index") -> (element=→"Display best fit parameters":dbl[])  [unwired: 1 in]
        n258 = local write "fits"(w716) -> ()
        n259 = for {
          N: w712 -> [_]
          tunnel: w667 -> [w814]
          tunnel: [w821] -> w685 mode=indexing
          tunnel: w715 -> [w819]
          tunnel: w681 -> [w818]
          tunnel: [w816] -> w680 mode=indexing
          tunnel: w679 -> [w815]
          tunnel: [w812] -> w678 mode=indexing
          tunnel: w668 -> [w811]
          tunnel: w667 -> [w809]
          tunnel: [w807] -> w666 mode=indexing
          i -> [w810]
          n260 = Index Array(array=w811, index (col)=w810) -> (element=w808:dbl[])  [unwired: 1 in]
          n261 = Index Array(array=w819, index (col)=w810) -> (element=w820:dbl[])  [unwired: 1 in]
          n262 = Index Array(array=w818, index (col)=w810) -> (element=w817:dbl[])  [unwired: 1 in]
          n263 = Index Array(array=w815, index (col)=w810) -> (element=w813:dbl[])  [unwired: 1 in]
          n264 = Bundle(w814, "Sorted Array out"=w820) -> (w821:cluster{dbl[], "Sorted Array out":dbl[]})  [unwired: 1 in]
          n265 = Bundle(w814, "reordered array"=w817) -> (w816:cluster{dbl[], "reordered array":dbl[]})  [unwired: 1 in]
          n266 = Bundle(w809, "reordered array"=w808) -> (w807:cluster{dbl[], "reordered array":dbl[]})  [unwired: 1 in]
          n267 = Bundle(w814, "Best Fit Parameters"=w813) -> (w812:cluster{dbl[], "Best Fit Parameters":dbl[]})  [unwired: 1 in]
        }
        "amplitudes" <- w680
        "widths" <- w678
        "position errors" <- w666
        n268 = local write "Restricted G"(w721) -> ()
        n269 = Index Array(array=w721, index="display index") -> (element=w677:cluster{dbl[], dbl[]})
        n270 = Index Array(array=w716, index="display index") -> (element=w676:cluster{dbl[], dbl[]})
        n271 = Unbundle(w677) -> (w673:dbl[], w675:dbl[])
        n272 = Unbundle(w676) -> (w674:dbl[])  [unwired: 1 out]
        n273 = Subtract(x=w675, y=w674) -> (x-y=w672:dbl[])
        n274 = call <vilib>:"Add State(s) to Queue__JKI_lib_State_Machine.vi"("State(s) in (\"\")"=w726) -> ("States Out"=w725:string)  [unwired: 14 in]
        n275 = local write "fits 2"(w685) -> ()
        n276 = Bundle(w673, w672) -> (w671:cluster{dbl[], dbl[]})  [unwired: 1 in]
        n277 = Index Array(array=w685, index #1="pair index 1", index #2="pair index 2") -> (element #1=w709:cluster{dbl[], "Sorted Array out":dbl[]}, element #2=w708:cluster{dbl[], "Sorted Array out":dbl[]})
        n278 = Index Array(array=w685, index #1="trion index 1", index #2="trion index 2", index #3="trion index 3") -> (element #1=w701:cluster{dbl[], "Sorted Array out":dbl[]}, element #2=w700:cluster{dbl[], "Sorted Array out":dbl[]}, element #3=w699:cluster{dbl[], "Sorted Array out":dbl[]})
        n279 = Unbundle(w709) -> (w706:dbl[], "Sorted Array out"=w684:dbl[])
        n280 = Unbundle(w708) -> ("Sorted Array out"=w683:dbl[])  [unwired: 1 out]
        n281 = Unbundle(w699) -> ("Sorted Array out"=w692:dbl[])  [unwired: 1 out]
        n282 = Unbundle(w700) -> ("Sorted Array out"=w693:dbl[])  [unwired: 1 out]
        n283 = Unbundle(w701) -> (w691:dbl[], "Sorted Array out"=w694:dbl[])
        n284 = Build Array(w677, w676, w671) -> (w722:cluster{dbl[], dbl[]}[])
        n285 = for {
          tunnel: w694 -> [w801] mode=indexing
          tunnel: w693 -> [w800] mode=indexing
          tunnel: w692 -> [w799] mode=indexing
          tunnel: [w797] -> w689 mode=indexing
          n286 = Build Array(w801, w800, w799) -> (w798:dbl[])
          n287 = call <vilib>:"Std Deviation and Variance.vi"("X"=w798) -> ("standard deviation"=w797:dbl)  [unwired: 1 in, 2 out]
        }
        n288 = for {
          tunnel: w684 -> [w796] mode=indexing
          tunnel: w683 -> [w795] mode=indexing
          tunnel: [w793] -> w682 mode=indexing
          n289 = Build Array(w796, w795) -> (w794:dbl[])
          n290 = call <vilib>:"Std Deviation and Variance.vi"("X"=w794) -> ("standard deviation"=w793:dbl)  [unwired: 1 in, 2 out]
        }
        n291 = local write "display fit"(w722) -> ()
        n292 = Array Subset(array=w706, index="display index", length="display length") -> (w696:dbl[])
        n293 = Array Subset(array=w682, index="display index", length="display length") -> (w705:dbl[])
        n294 = Bundle(w696, w705) -> (→"pair":cluster{dbl[], dbl[]})  [unwired: 1 in]
        n295 = Array Subset(array=w691, index="display index 2", length="display length 2") -> (w690:dbl[])
        n296 = Array Subset(array=w689, index="display index 2", length="display length 2") -> (w688:dbl[])
        n297 = Bundle(w690, w688) -> (→"trion":cluster{dbl[], dbl[]})  [unwired: 1 in]
        "done" <- TRUE ("done")
      }
    }
  }
  n298 = disable-structure shown="Disabled" {
    frame Disabled {
      # "fitting sanity check"
      n299 = call "string model.vi"() -> ("model"=w827:string, "Parameters"=w824:string[])  [unwired: 9 in, 1 out]
      n300 = Unbundle() -> (w830)  [unwired: 1 in, 1 out]
      n301 = Concatenate Strings("y=" ("string"), w827, ";" ("string")) -> (w828:string)
      n302 = for {
        tunnel: _ -> [w841]
        tunnel: w830 -> [w842]
        tunnel: w828 -> [w839]
        tunnel: "x" ("x") -> [w838]
        tunnel: w824 -> [w837]
        tunnel: string[] ["y"] ("Variables Output") -> [w835]
        tunnel: [w833] -> w829 mode=indexing
        tunnel: _ -> [w832]
        tunnel: [w831] -> _
        n303 = Build Array (concatenate)(w838, w837) -> (w836:string[])
        n304 = Build Array (concatenate)(w842, w841) -> (w840:void[])
        n305 = call <vilib>:"Eval Formula Node.vi"("Variables Input"=w836, "Input Values"=w840, "Variables Output"=w835, "formula"=w839, "error in (no error)"=w832) -> ("Output Values"=w834:dbl[], "error out"=w831:errorcluster)
        n306 = Index Array(array=w834) -> (element=w833:dbl)  [unwired: 1 in]
      }
      n307 = Bundle(w830, w829) -> ()  [unwired: 1 in, 1 out]
    }
    frame Enabled {
    }
  }
